vi "Pass.vi"(7 "Description":string, 8 "error in (no error)":errorcluster, 9 "Message":string, 11 "LUnit Test Case In":refnum<class "LUnit Test Case.lvclass">) -> (0 "error out":errorcluster, 3 "LUnit Test Case Out":refnum<class "LUnit Test Case.lvclass">)   [LabVIEW 2020, in "LUnit Test Case.lvclass"]
doc: "Generates a pass result for the calling test method. A description and message may be provided."
uses:
  LUnit Test Case.lvclass
  Result Types/Assertion Result/Public/TypeDefs/Assertion Type.ctl
  LUnit Test Case.lvclass/LUnit Test Case.ctl
  Result Types/Assertion Result/Public/TypeDefs/Status.ctl
  Result Types/Case Result/Public/Record Assertion Result.vi
  Result Types/Method Result/Public/Aggregate Assertion Results.vi
  Result Types/Method Result/Private/Merge Status.vi
  Result Types/Method Result/Private/Concatenate result strings.vi
  Result Types/Assertion Result/Assertion Result.lvlib
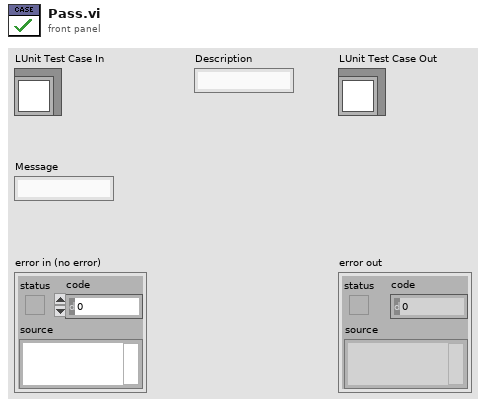
[diagram p1: front panel]
types:
  T1 = typedef "Assertion Result.lvlib/Assertion Type.ctl" = enum16{"None", "Pass", "Fail", "Skip", "Pass if Equal", "Fail if Equal", "Pass if Error", "Fail if Error", "Pass if", "Fail if"}
  T2 = typedef "Assertion Result.lvlib/Assertion Result type.ctl" = cluster{"Status":T3, "Message":string, "Description":string, "Assertion Type":T1}
  T3 = typedef "Assertion Result.lvlib/Status.ctl" = enum16{"Pass", "Fail", "Error", "Skipped", "Setup Error", "Broken", "Teardown Error"}
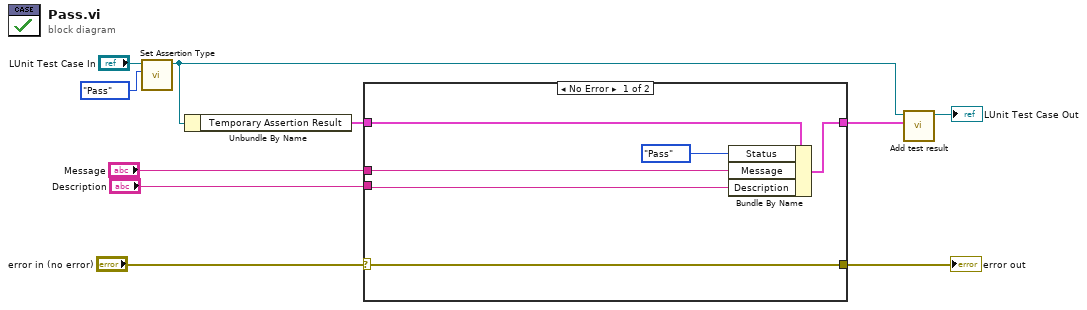
[diagram p0: block diagram]
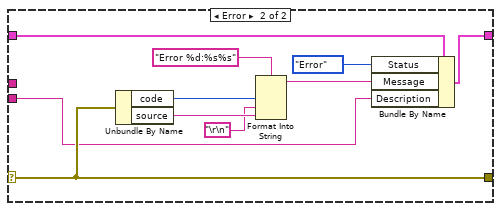
[diagram p2: hidden frame]
diagram:
  n1 = call "Set Assertion Type.vi"("Assertion Type"=Assertion_Type."Pass", "LUnit Test Case In"="LUnit Test Case In") -> ("LUnit Test Case Out"=w6:refnum<class "LUnit Test Case.lvclass">)  [unwired: 9 in]
  n2 = Unbundle By Name(w6) -> ("Temporary Assertion Result"=w9:T2)
  n3 = case shown="No Error" "error in (no error)" {
    selector: "error in (no error)" -> [w14 w22]
    tunnel: w9 -> [w16 w18]
    tunnel: [w15 w19] -> w1
    tunnel: [w14 w22] -> w4
    tunnel: "Message" -> [w13 _]
    tunnel: "Description" -> [w11 w17]
    frame No Error {
      n4 = Bundle By Name(cluster=w16, "Status"=Status."Pass", "Message"=w13, "Description"=w11) -> (w15:T2)
    }
    frame Error {
      n5 = Unbundle By Name(w22) -> ("code"=w26:i32, "source"=w24:string)
      n6 = Format Into String(format string="Error %d:%s%s", w26, "\r\n", w24) -> (resulting string=w25:string)  [unwired: 2 in, 1 out]
      n7 = Bundle By Name(cluster=w18, "Status"=Status."Error", "Message"=w25, "Description"=w17) -> (w19:T2)
    }
  }
  "error out" <- w4
  n8 = call "Add test result.vi"("Test Result"=w1, "LUnit Test Case In"=w6) -> ("LUnit Test Case Out"=→"LUnit Test Case Out":refnum<class "LUnit Test Case.lvclass">)  [unwired: 9 in]
